vi "set_unit_mode.vi"(8 "error in (no error)":errorcluster caption="错误输入（无错误）", 10 "unit mode":T1, 11 "OneMotion输入":refnum<class "OneMotion.lvclass">) -> (0 "error out":errorcluster caption="错误输出", 3 "OneMotion输出":refnum<class "OneMotion.lvclass">)   [LabVIEW 2016, in "MotionControl_UFO_3DOF.lvlib" / "OneMotion.lvclass"]
uses:
  <userlib>/MotionControl_UFO_3DOF/OneMotion/OneMotion.lvclass
  <userlib>/MotionControl_UFO_3DOF/OneMotion/unit mode.ctl
  <userlib>/MotionControl_UFO_3DOF/OneMotion/OneMotion.lvclass/OneMotion.ctl
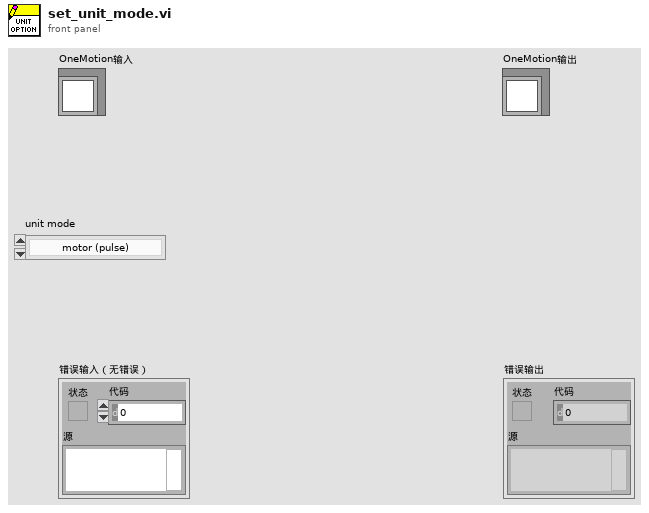
[diagram p1: front panel]
types:
  T1 = typedef "MotionControl_UFO_3DOF.lvlib/OneMotion.lvclass/unit mode.ctl" = enum16{"motor (pulse)", "linear (mm) or radial (degree)"}
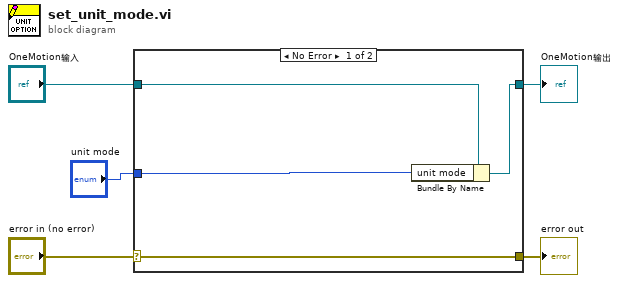
[diagram p0: block diagram]
diagram:
  n1 = case shown="No Error" "error in (no error)" {
    selector: "error in (no error)" -> [w9 w10]
    tunnel: [w9 w10] -> w4
    tunnel: [w7 w11] -> w2
    tunnel: "OneMotion输入" -> [w8 w11]
    tunnel: "unit mode" -> [w6 _]
    frame No Error {
      n2 = Bundle By Name(cluster=w8, "unit mode"=w6) -> (w7:refnum<class "OneMotion.lvclass">)
    }
    frame Error {
    }
  }
  "error out" <- w4
  "OneMotion输出" <- w2
